vi "Angle in defense.vi"(6 "Forward Right US":dbl, 9 "Back Left US":dbl, 10 "Back Right US":dbl, 11 "Forward Left US":dbl) -> (1 "d":dbl, 2 "AlphaL":dbl, 3 "AlphaR":dbl)   [LabVIEW 2016]
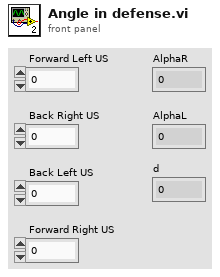
[diagram p1: front panel]
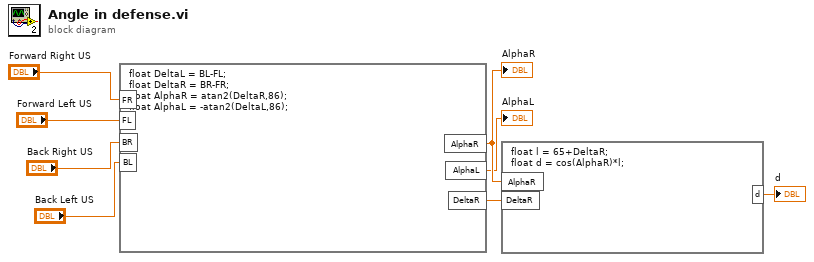
[diagram p0: block diagram]
diagram:
  n1 = formula code="float DeltaL = BL-FL;\nfloat DeltaR = BR-FR;\nfloat AlphaR = atan2(DeltaR,86);\nfloat AlphaL = -atan2(DeltaL,86);"("FR"="Forward Right US", "FL"="Forward Left US", "BR"="Back Right US", "BL"="Back Left US") -> ("AlphaR"=w4:dbl, "AlphaL"=→"AlphaL":dbl, "DeltaR"=w2:dbl)
  "AlphaR" <- w4
  n2 = formula code="float l = 65+DeltaR;\nfloat d = cos(AlphaR)*l;"("AlphaR"=w4, "DeltaR"=w2) -> ("d"=→"d":dbl)
